vi "Memory.Pointer.Offset to Address.Safe.vi"(8 "error in (no error)":errorcluster, 10 "offset":u64 format="%d bytes", 11 "Pointer in":refnum<class "Memory.Pointer.Void.lvclass">) -> (0 "error out":errorcluster, 2 "address":u64 format="%016x", 3 "Pointer out":refnum<class "Memory.Pointer.Void.lvclass">)   [LabVIEW 2016, in "LabVIEW Memory Manager.lvlib" / "Memory.Pointer.Void.lvclass"]
uses:
  Memory.Pointer.Void.lvclass
  Memory.Pointer.Void.lvclass/Memory.Pointer.Void.ctl
  Memory.Pointer.Get Size.vi
  Memory.Pointer.Get Address.vi
  Memory.Pointer.Error Handling.Out of Range.vi
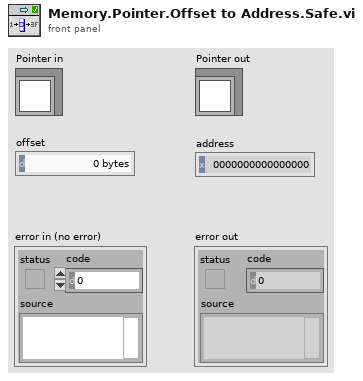
[diagram p1: front panel]
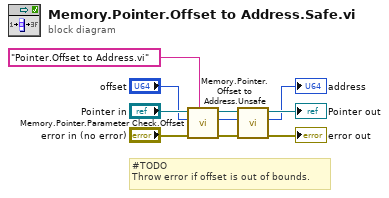
[diagram p0: block diagram]
diagram:
  # "#TODO\nThrow error if offset is out of bounds."
  n1 = call "Memory.Pointer.Parameter Check.Offset.vi"("calling vi name"="Pointer.Offset to Address.vi", "error in (no error)"="error in (no error)", "offset"="offset", "Pointer in"="Pointer in") -> ("error out"=w5:errorcluster, "offset out"=w2:u64, "Pointer out"=w6:refnum<class "Memory.Pointer.Void.lvclass">)  [unwired: 5 in]
  n2 = call "Memory.Pointer.Offset to Address.Unsafe.vi"("error in (no error)"=w5, "offset"=w2, "Pointer in"=w6) -> ("error out"=→"error out":errorcluster, "address"=→"address":u64, "Pointer out"=→"Pointer out":refnum<class "Memory.Pointer.Void.lvclass">)  [unwired: 6 in]
